vi "Patrick GDSII.vi"() -> ()   [LabVIEW 2019]
panel:
  out "Record 2":T1(array[cluster])
  out "converted":T2(array[cluster])
  out "Records":T3(array[cluster]) {"byte 3 (Record Type)" format="%04x"; "byte 4 (Data Type)" format="%04x"}
  in  "GDSII file path (use dialog)":path
  out "data":u8[](array[numeric])
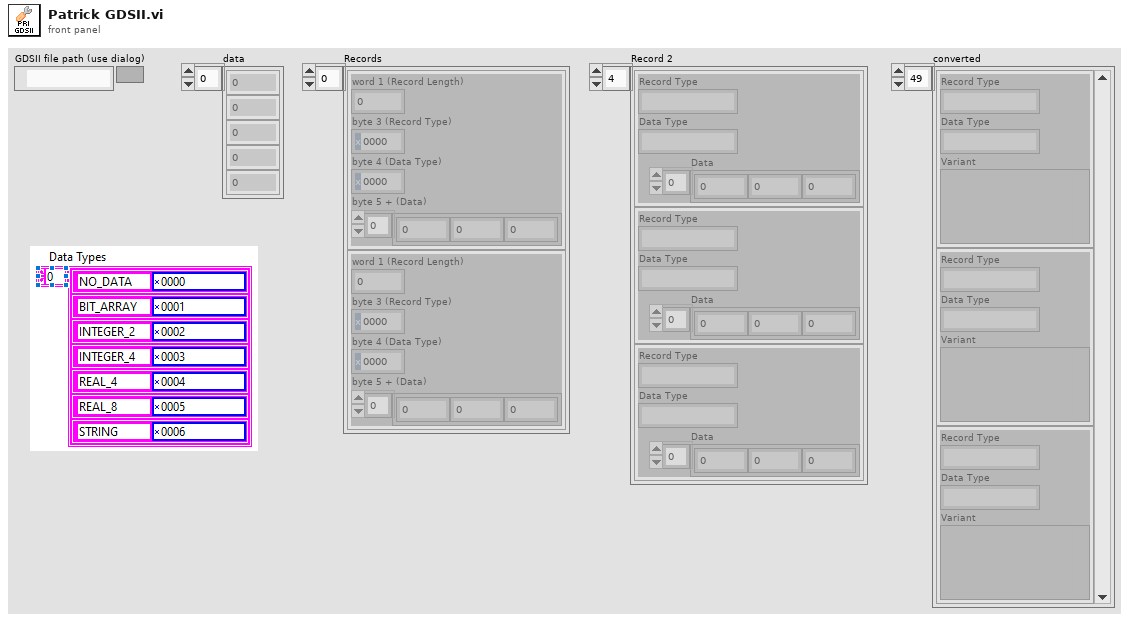
[diagram p1: front panel]
types:
  T1 = cluster{"Record Type":string, "Data Type":string, "Data":u8[]}[]
  T2 = cluster{"Record Type":string, "Data Type":string, "Variant":variant}[]
  T3 = cluster{"word 1 (Record Length)":u16, "byte 3 (Record Type)":u8, "byte 4 (Data Type)":u8, "byte 5 + (Data)":u8[]}[]
  T4 = cluster{"word 1 (Record Length)":u16, "byte 3 (Record Type)":u8, "byte 4 (Data Type)":u8, "byte 5 + (Data)":u8[]}
  T5 = cluster{"Record Type":string, "Data Type":string, "Data":u8[]}
  T6 = cluster{"Record Type":string, "Data Type":string, "Variant":variant}
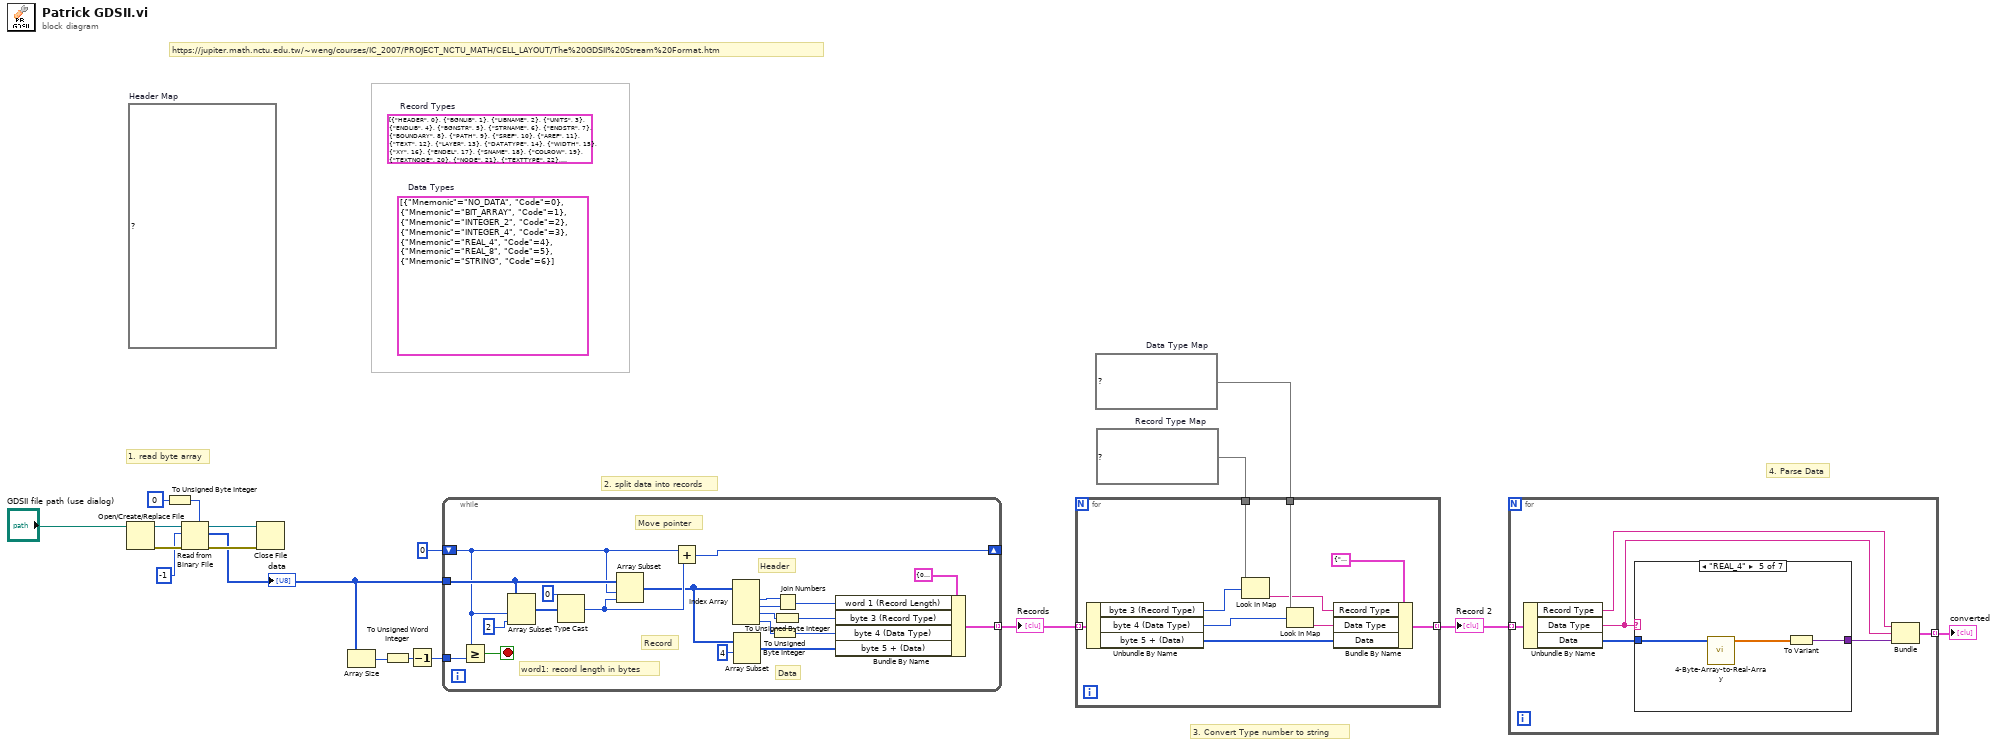
[diagram p0: block diagram]
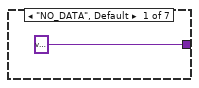
[diagram p2: hidden frame]
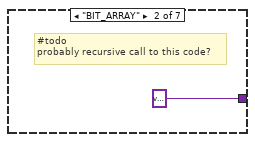
[diagram p3: hidden frame]
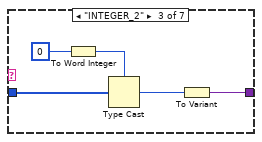
[diagram p4: hidden frame]
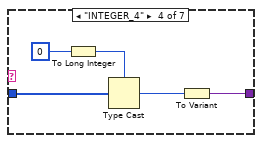
[diagram p5: hidden frame]
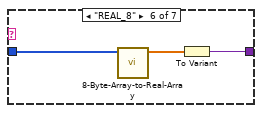
[diagram p6: hidden frame]
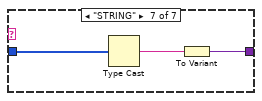
[diagram p7: hidden frame]
diagram:
  w5 = map{u8, string} {0="NO_DATA", 1="BIT_ARRAY", 2="INTEGER_2", 3="INTEGER_4", 4="REAL_4", 5="REAL_8", 6="STRING"}  # Data Type Map
  w6 = map{u8, string} {0="HEADER", 1="BGNLIB", 2="LIBNAME", 3="UNITS", 4="ENDLIB", 5="BGNSTR", 6="STRNAME", 7="ENDSTR", 8="BOUNDARY", 9="PATH", 10="SREF", 11="AREF", 12="TEXT", 13="LAYER", 14="DATATYPE", 15="WIDTH", 16="XY", 17="ENDEL", 18="SNAME", 19="COLROW", 20="TEXTNODE", 21="NODE", 22="TEXTTYPE", 23="PRESENTATION", 24="SPACING", 25="STRING", 26="STRANS", 27="MAG", 28="ANGLE", 29="UINTEGER", 30="USTRING", 31="REFLIBS", 32="FONTS", 33="PATHTYPE", 34="GENERATIONS", 35="ATTRTABLE", 36="STYPTABLE", 37="STRTYPE", 38="ELFLAGS", 39="ELKEY", 40="LINKTYPE", 41="LINKKEYS", 42="NODETYPE", 43="PROPATTR", 44="PROPVALUE", 45="BOX", 46="BOXTYPE", 47="PLEX", 48="BGNEXTN", 49="ENDTEXTN", 50="TAPENUM", 51="TAPECODE", 52="STRCLASS", 53="RESERVED", 54="FORMAT", 55="MASK", 56="ENDMASKS", 57="LIBDIRSIZE", 58="SRFNAME", 59="LIBSECUR"}  # Record Type Map
  (unwired) cluster{"Mnemonic":string, "Code":u8}[] [{"Mnemonic"="NO_DATA", "Code"=0}, {"Mnemonic"="BIT_ARRAY", "Code"=1}, {"Mnemonic"="INTEGER_2", "Code"=2}, {"Mnemonic"="INTEGER_4", "Code"=3}, {"Mnemonic"="REAL_4", "Code"=4}, {"Mnemonic"="REAL_8", "Code"=5}, {"Mnemonic"="STRING", "Code"=6}]  # Data Types
  (unwired) cluster{"Mnemonic":string, "Code":u8}[] [{"Mnemonic"="HEADER", "Code"=0}, {"Mnemonic"="BGNLIB", "Code"=1}, {"Mnemonic"="LIBNAME", "Code"=2}, {"Mnemonic"="UNITS", "Code"=3}, {"Mnemonic"="ENDLIB", "Code"=4}, {"Mnemonic"="BGNSTR", "Code"=5}, {"Mnemonic"="STRNAME", "Code"=6}, {"Mnemonic"="ENDSTR", "Code"=7}, {"Mnemonic"="BOUNDARY", "Code"=8}, {"Mnemonic"="PATH", "Code"=9}, {"Mnemonic"="SREF", "Code"=10}, {"Mnemonic"="AREF", "Code"=11}, {"Mnemonic"="TEXT", "Code"=12}, {"Mnemonic"="LAYER", "Code"=13}, {"Mnemonic"="DATATYPE", "Code"=14}, {"Mnemonic"="WIDTH", "Code"=15}, {"Mnemonic"="XY", "Code"=16}, {"Mnemonic"="ENDEL", "Code"=17}, {"Mnemonic"="SNAME", "Code"=18}, {"Mnemonic"="COLROW", "Code"=19}, {"Mnemonic"="TEXTNODE", "Code"=20}, {"Mnemonic"="NODE", "Code"=21}, {"Mnemonic"="TEXTTYPE", "Code"=22}, {"Mnemonic"="PRESENTATION", "Code"=23}, {"Mnemonic"="SPACING", "Code"=24}, {"Mnemonic"="STRING", "Code"=25}, {"Mnemonic"="STRANS", "Code"=26}, {"Mnemonic"="MAG", "Code"=27}, {"Mnemonic"="ANGLE", "Code"=28}, {"Mnemonic"="UINTEGER", "Code"=29}, {"Mnemonic"="USTRING", "Code"=30}, {"Mnemonic"="REFLIBS", "Code"=31}, {"Mnemonic"="FONTS", "Code"=32}, {"Mnemonic"="PATHTYPE", "Code"=33}, {"Mnemonic"="GENERATIONS", "Code"=34}, {"Mnemonic"="ATTRTABLE", "Code"=35}, {"Mnemonic"="STYPTABLE", "Code"=36}, {"Mnemonic"="STRTYPE", "Code"=37}, {"Mnemonic"="ELFLAGS", "Code"=38}, {"Mnemonic"="ELKEY", "Code"=39}, {"Mnemonic"="LINKTYPE", "Code"=40}, {"Mnemonic"="LINKKEYS", "Code"=41}, {"Mnemonic"="NODETYPE", "Code"=42}, {"Mnemonic"="PROPATTR", "Code"=43}, {"Mnemonic"="PROPVALUE", "Code"=44}, {"Mnemonic"="BOX", "Code"=45}, {"Mnemonic"="BOXTYPE", "Code"=46}, {"Mnemonic"="PLEX", "Code"=47}, {"Mnemonic"="BGNEXTN", "Code"=48}, {"Mnemonic"="ENDTEXTN", "Code"=49}, {"Mnemonic"="TAPENUM", "Code"=50}, {"Mnemonic"="TAPECODE", "Code"=51}, {"Mnemonic"="STRCLASS", "Code"=52}, {"Mnemonic"="RESERVED", "Code"=53}, {"Mnemonic"="FORMAT", "Code"=54}, {"Mnemonic"="MASK", "Code"=55}, {"Mnemonic"="ENDMASKS", "Code"=56}, {"Mnemonic"="LIBDIRSIZE", "Code"=57}, {"Mnemonic"="SRFNAME", "Code"=58}, {"Mnemonic"="LIBSECUR", "Code"=59}]  # Record Types
  (unwired) map{i16, string} {2="HEADER", 258="BGNLIB", 518="LIBNAME", 773="UNITS", 1024="ENDLIB", 1282="BGNSTR", 1542="STRNAME", 1792="ENDSTR", 2048="BOUNDARY", 2304="PATH", 2560="SREF", 2816="AREF", 3072="TEXT", 3330="LAYER", 3586="DATATYPE", 3843="WIDTH", 4099="XY", 4352="ENDEL", 4614="SNAME", 4866="COLROW", 5376="NODE", 5634="TEXTTYPE", 5889="PRESENTATION", 6406="STRING", 6657="STRANS", 6917="MAG", 7173="ANGLE", 7942="REFLIBS", 8198="FONTS", 8450="PATHTYPE", 8706="GENERATIONS", 8966="ATTRTABLE", 9729="ELFLAGS", 10754="NODETYPE", 11010="PROPATTR", 11270="PROPVALUE", 11520="BOX", 11778="BOXTYPE", 12035="PLEX", 12802="TAPENUM", 13059="TAPECODE", 13826="FORMAT", 14086="MASK", 14336="ENDMASKS"}  # Header Map
  # "4. Parse Data"
  # "3. Convert Type number to string"
  # "https://jupiter.math.nctu.edu.tw/~weng/courses/IC_2007/PROJECT_NCTU_MATH/CELL_LAYOUT/The%20GDSII%20Stream%20Format.htm"
  # "2. split data into records"
  # "1. read byte array"
  n1 = Open/Create/Replace File(file path (use dialog)="GDSII file path (use dialog)") -> (refnum out=w18:refnum<file>, error out=w16:errorcluster)  [unwired: 5 in, 1 out]
  n2 = To Unsigned Byte Integer(number=u8 0) -> (unsigned 8bit integer=w1:u8)
  n3 = Read from Binary File(5:w1, 8:w16, 10:-1 ("count (1)"), 11:w18) -> (0:w15:errorcluster, 2:w10:u8[], 3:w17:refnum<file>)  [unwired: 2 in, 1 out]
  "data" <- w10
  n4 = Close File(refnum=w17, error in=w15) -> ()  [unwired: 2 out]
  n5 = Array Size(array=w10) -> (size(s)=w9:i32)
  n6 = To Unsigned Word Integer(number=w9) -> (unsigned 16bit integer=w8:u16)
  n7 = Decrement(x=w8) -> (x-1=w11:u16)
  n8 = while {
    tunnel: w10 -> [w35]
    shift-right: [w33] -> _
    shift-left: u16 0 -> [w34]
    tunnel: w11 -> [w38]
    tunnel: [w28] -> w7 mode=indexing
    stop <- w39 stop-if-true
    # "Move pointer"
    # "Data"
    # "Header"
    # "Record"
    # "word1: record length in bytes"
    n9 = Greater Or Equal?(x=w34, y=w38) -> (x >= y?=w39:bool)
    n10 = Array Subset(array=w35, index=w34, length=2 ("length (rest)")) -> (w36:u8[])
    n11 = Type Cast(type=u16 0, x=w36) -> (*(type *) &x=w31:u16)
    n12 = Array Subset(array=w35, index=w34, length=w31) -> (w26:u8[])
    n13 = Add(x=w34, y=w31) -> (x+y=w33:u16)
    n14 = Index Array(array=w26) -> (element #1=w25:u8, element #2=w24:u8, element #3=w19:u8, element #4=w20:u8)  [unwired: 4 in]
    n15 = Array Subset(array=w26, index=4) -> (w29:u8[])  [unwired: 1 in]
    n16 = To Unsigned Byte Integer(number=w20) -> (unsigned 8bit integer=w21:u8)
    n17 = To Unsigned Byte Integer(number=w19) -> (unsigned 8bit integer=w22:u8)
    n18 = Join Numbers(hi=w25, lo=w24) -> ((hi.lo)=w23:u16)
    n19 = Bundle By Name(cluster=T4 {"word 1 (Record Length)"=0, "byte 3 (Record Type)"=0, "byte 4 (Data Type)"=0, "byte 5 + (Data)"=[]}, "word 1 (Record Length)"=w23, "byte 3 (Record Type)"=w22, "byte 4 (Data Type)"=w21, "byte 5 + (Data)"=w29) -> (w28:T4)
  }
  "Records" <- w7
  n20 = for {
    tunnel: w7 -> [w49] mode=indexing
    tunnel: w6 -> [w48]
    tunnel: w5 -> [w47]
    tunnel: [w40] -> w4 mode=indexing
    n21 = Unbundle By Name(w49) -> ("byte 3 (Record Type)"=w41:u8, "byte 4 (Data Type)"=w46:u8, "byte 5 + (Data)"=w42:u8[])
    n22 = Look In Map(map=w48, key=w41) -> (value=w44:string)  [unwired: 1 in, 1 out]
    n23 = Look In Map(map=w47, key=w46) -> (value=w43:string)  [unwired: 1 in, 1 out]
    n24 = Bundle By Name(cluster=T5 {"Record Type"="", "Data Type"="", "Data"=[]}, "Record Type"=w44, "Data Type"=w43, "Data"=w42) -> (w40:T5)
  }
  "Record 2" <- w4
  n25 = for {
    tunnel: w4 -> [w55] mode=indexing
    tunnel: [w52] -> w3 mode=indexing
    n26 = Unbundle By Name(w55) -> ("Record Type"=w51:string, "Data Type"=w50:string, "Data"=w54:u8[])
    n27 = case shown="\"REAL_4\"" w50 {
      tunnel: w54 -> [_ _ w62 w65 w69 w72 w76]
      tunnel: [variant ("Variant") variant ("Variant") w59 w64 w70 w73 w74] -> w53
      frame "NO_DATA", Default {
      }
      frame "BIT_ARRAY" {
        # "#todo\nprobably recursive call to this code?"
      }
      frame "INTEGER_2" {
        n28 = To Word Integer(number=i16 0) -> (16bit integer=w58:i16)
        n29 = Type Cast(type=w58, x=w62) -> (*(type *) &x=w60:i16)
        n30 = To Variant(anything=w60) -> (Variant=w59:variant)
      }
      frame "INTEGER_4" {
        n31 = To Long Integer(number=0) -> (32bit integer=w63:i32)
        n32 = Type Cast(type=w63, x=w65) -> (*(type *) &x=w66:i32)
        n33 = To Variant(anything=w66) -> (Variant=w64:variant)
      }
      frame "REAL_4" {
        n34 = call "4-Byte-Array-to-Real-Array.vi"("Data"=w69) -> ("Array of Values"=w68:dbl[])  [unwired: 10 in]
        n35 = To Variant(anything=w68) -> (Variant=w70:variant)
      }
      frame "REAL_8" {
        n36 = call "8-Byte-Array-to-Real-Array.vi"("Data"=w72) -> ("Array of Values"=w71:dbl[])  [unwired: 10 in]
        n37 = To Variant(anything=w71) -> (Variant=w73:variant)
      }
      frame "STRING" {
        n38 = Type Cast(x=w76) -> (*(type *) &x=w75:string)  [unwired: 1 in]
        n39 = To Variant(anything=w75) -> (Variant=w74:variant)
      }
    }
    n40 = Bundle("Record Type"=w51, "Data Type"=w50, "Variant"=w53) -> (w52:T6)  [unwired: 1 in]
  }
  "converted" <- w3
